vi "headligthsAdjusterVI.vi"() -> ()   [LabVIEW 2021]
uses:
  <vilib>/Instr/_visa.llb/VISA Configure Serial Port (Instr).vi
panel:
  out "Waveform Graph":dbl[](graph)
  out "Waveform Chart":dbl(graph)
  in  "VISA resource name":refnum<visa-resource-name>
  out "Proximity":dbl
  out "String":string
  in  "stop":bool
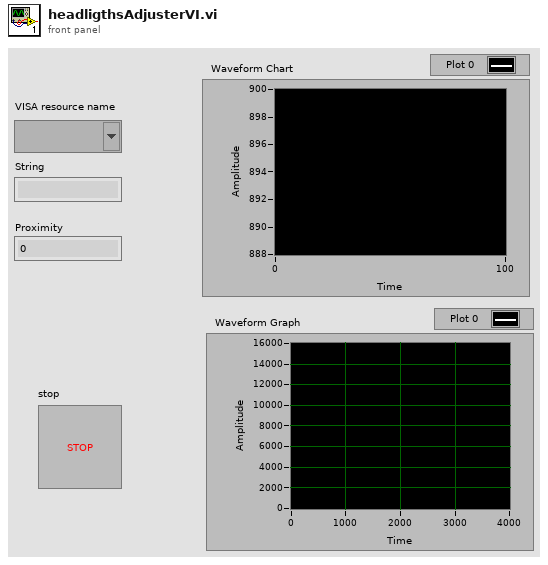
[diagram p1: front panel]
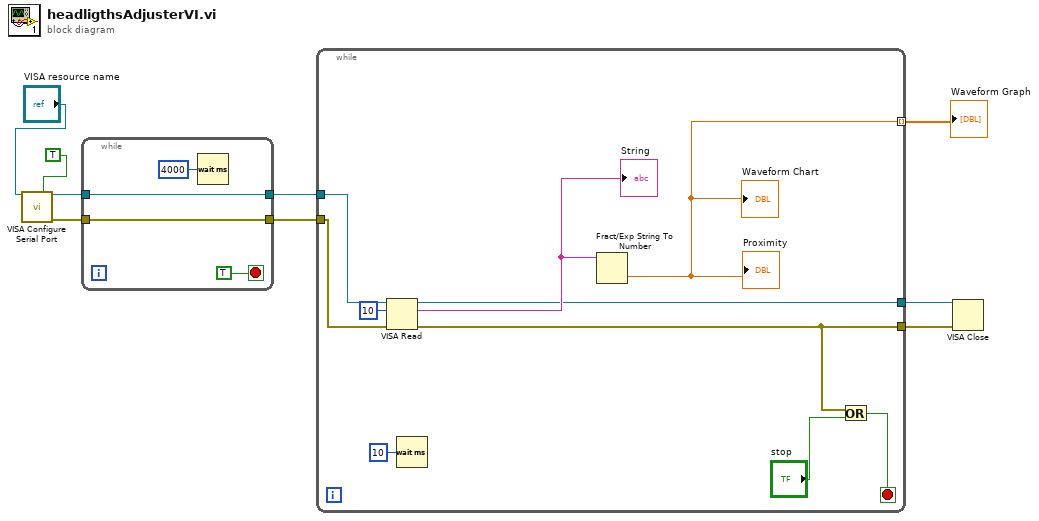
[diagram p0: block diagram]
diagram:
  n1 = call-poly "VISA Configure Serial Port"("VISA resource name"="VISA resource name", "Enable Termination\nChar (T)"=TRUE ("Enable Termination\nChar (T)")) -> ("VISA resource name out"=w8:refnum<visa-resource-name>, "error out"=w7:errorcluster)  [unwired: 12 in]
  n2 = while {
    tunnel: w8 -> [w11]
    tunnel: [w11] -> w6
    tunnel: w7 -> [w10]
    tunnel: [w10] -> w5
    stop <- TRUE stop-if-true
    n3 = Wait (ms)(milliseconds to wait=u32 4000) -> ()  [unwired: 1 out]
  }
  n4 = while {
    tunnel: w6 -> [w17]
    tunnel: w5 -> [w18]
    tunnel: [w20] -> w3
    tunnel: [w15] -> w2
    tunnel: [w14] -> w1 mode=indexing
    stop <- w21 stop-if-true
    n5 = VISA Read(VISA resource name=w17, byte count=u32 10, error in (no error)=w18) -> (VISA resource name out=w15:refnum<visa-resource-name>, read buffer=w16:string, error out=w20:errorcluster)  [unwired: 1 out]
    "String" <- w16
    n6 = Wait (ms)(milliseconds to wait=u32 10) -> ()  [unwired: 1 out]
    n7 = Fract/Exp String To Number(string=w16) -> (number=w14:dbl)  [unwired: 3 in, 1 out]
    "Proximity" <- w14
    "Waveform Chart" <- w14
    n8 = Or(x=w20, y="stop") -> (x .or. y?=w21:bool)
  }
  "Waveform Graph" <- w1
  n9 = VISA Close(VISA resource name=w2, error in (no error)=w3) -> ()  [unwired: 1 out]
